vi "test_DAQ_MG090622Camera.vi"() -> ()   [LabVIEW 2010, in "DAQ_MG090622Camera.lvclass"]
uses:
  DAQ_MG090622Camera.lvclass
  GenericDAQ/GenericDAQ/GenericDAQ.lvclass
  main/labview_source/type_definitions/enumerations/run_mode_enum.ctl
  main/labview_source/type_definitions/clusters/controls_refs.ctl
  common/classes/ErrorController/ErrorController/ErrorController.lvclass
panel:
  out "error controller loaded?":bool
  in  "user":string(combo)
  in  "duration":dbl[unit]=1.0
  in  "run mode":T1
  in  "start button":bool
  in  "createButton":bool
  in  "configuration name":string(combo)
  in  "stop":bool
  # "Test Suite for DAQ_MG090622Camera"
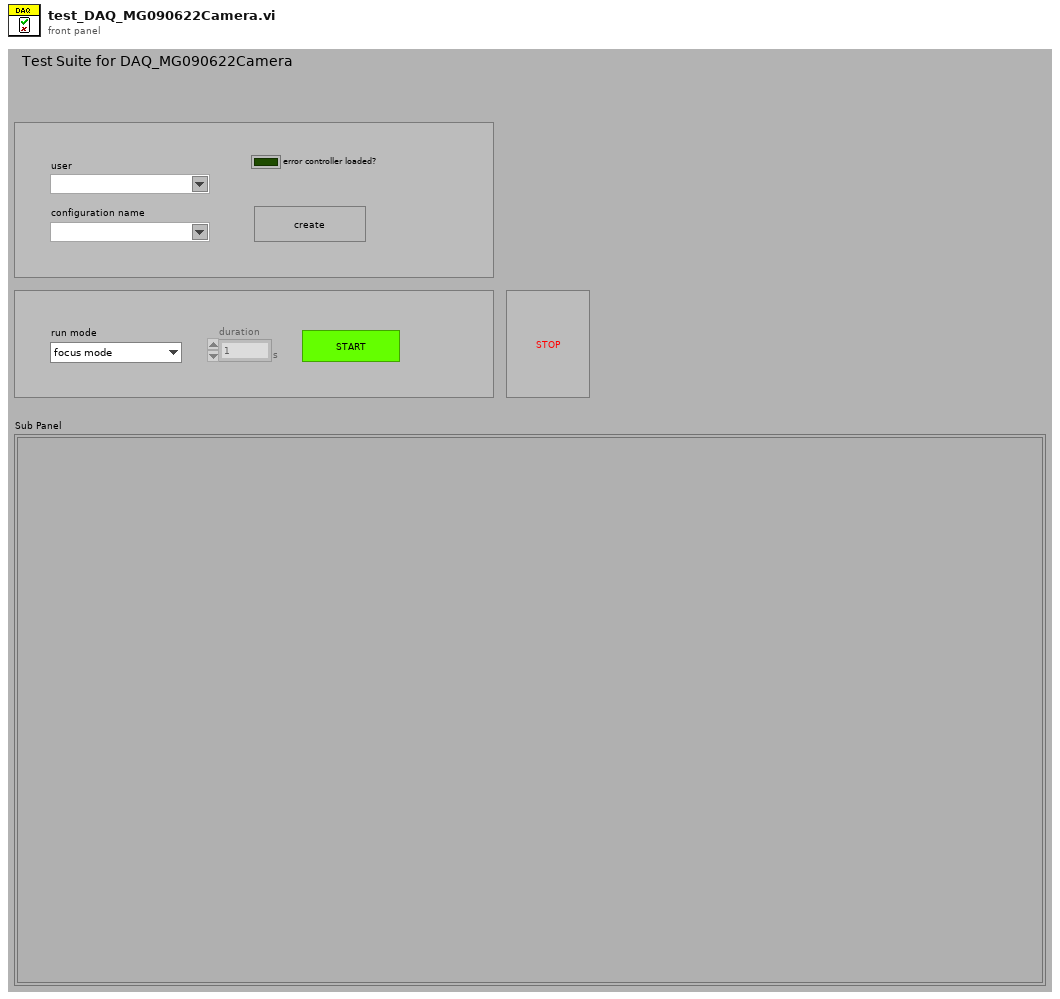
[diagram p1: front panel]
types:
  T1 = typedef "run_mode_enum.ctl" = enum16{"focus mode", "single sweep mode", "experiment mode"}
  T2 = typedef "controls_refs.ctl" = cluster{"scan start button":refnum<vi>, "tabs":cluster{"main":refnum<vi>, "settings":refnum<vi>}, "subpanels":cluster{"imagingMode":refnum<vi>, "scanHead":refnum<vi>, "display":refnum<vi>, "experimentController":refnum<vi>, "instrument":refnum<vi>, "stage":refnum<vi>, "stimulator":refnum<vi>, "dataCollection":refnum<vi>, "analyser":refnum<vi>, "daq":refnum<vi>, "imageAssembler":refnum<vi>}, "drop-downs":cluster{"run mode":refnum<vi>, "imagingMode":refnum<vi>, "experimentalController":refnum<vi>, "objective":refnum<vi>}, "status lights":cluster{"experimentController":refnum<vi>, "imagingMode":refnum<vi>, "scanHead":refnum<vi>, "daq":refnum<vi>, "imageAssembler":refnum<vi>, "dataCollection":refnum<vi>, "display":refnum<vi>, "analyser":refnum<vi>, "stage":refnum<vi>, "stimulator":refnum<vi>, "instrument":refnum<vi>}, "message":refnum<vi>, "stimulator enabled?":refnum<vi>, "saving":cluster{"data folder path":refnum<vi>, "file base name":refnum<vi>, "notebook":refnum<vi>}, "progress bar":refnum<vi>, "update icon":refnum<vi>, "title":refnum<vi>, "main vi":refnum<vi>, "user":refnum<vi>, "exit_button":refnum<vi>, "CPU usage %":refnum<vi>}
  T3 = typedef "plugin_specification.ctl" = cluster{"class path":string, "configuration":string, "label":string, "settings name":string}
  T4 = typedef "GenericToplevelComponent.lvclass/common_trigger_enum.ctl" = enum16{"NULL", "initialise", "terminate", "fetch command", "fetch data", "attach observer", "register as observer", "detach observer", "acknowledge", "start", "stop", "sweep started", "sweep finished", "experiment started", "experiment stopped"}
  T5 = enum8{"Enabled", "Disabled", "Disabled and Grayed Out"}
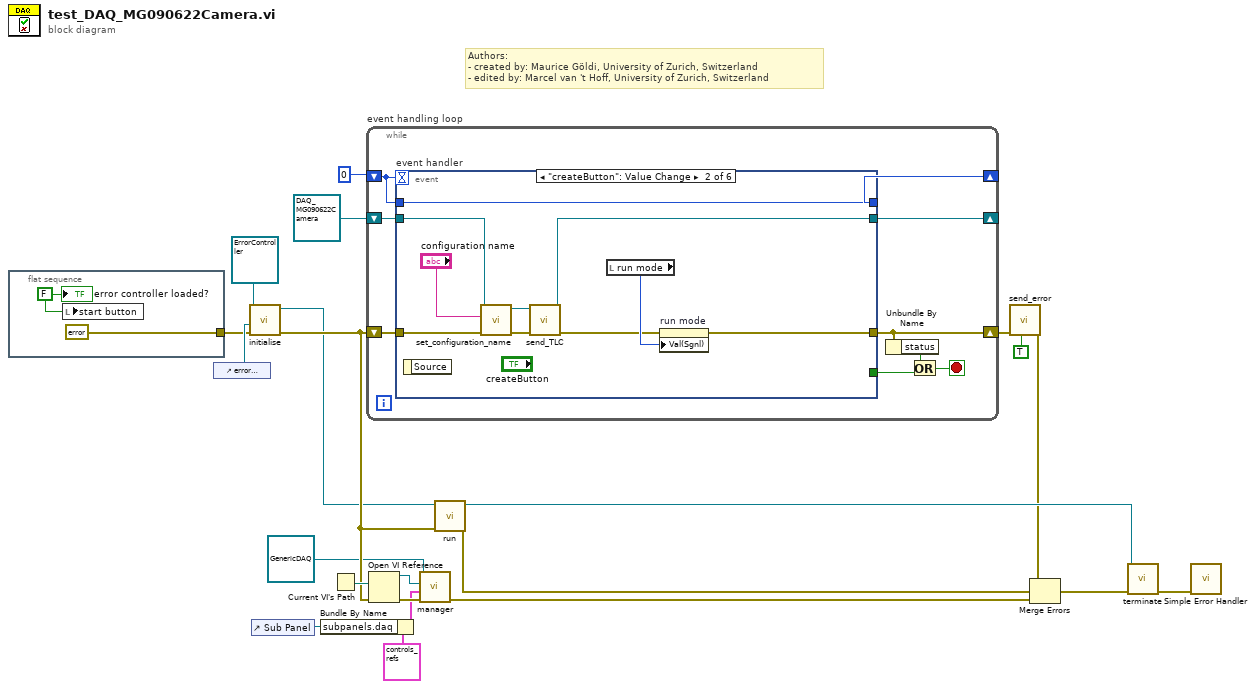
[diagram p0: block diagram]
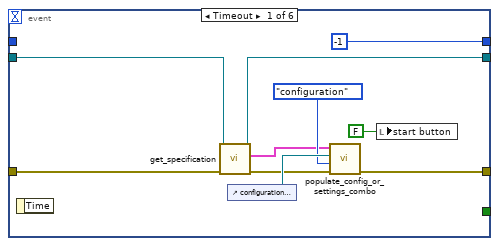
[diagram p2: hidden frame]
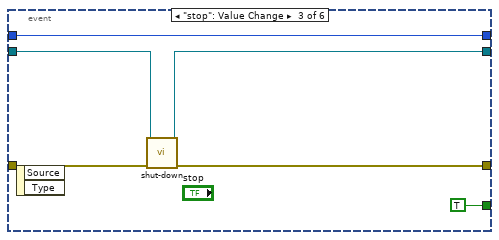
[diagram p3: hidden frame]
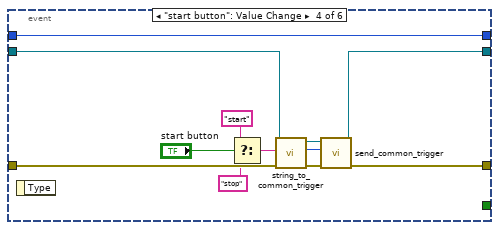
[diagram p4: hidden frame]
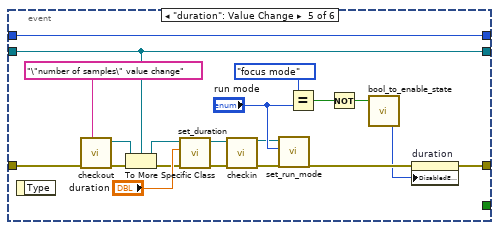
[diagram p5: hidden frame]
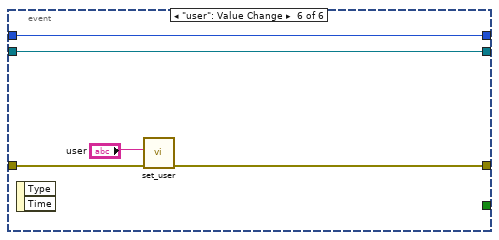
[diagram p6: hidden frame]
diagram:
  # "Authors: \n- created by: Maurice Göldi, University of Zurich, Switzerland\n- edited by: Marcel van 't Hoff, University of Zurich, Switzerland"
  n1 = flat-sequence {
    tunnel: [errorcluster {"status"=FALSE, "code"=0, "source"=""} ("error in (no error)")] -> w2
    frame #0 {
      w23 = FALSE ("error controller loaded?")
      n2 = local write "start button"(w23) -> ()
      "error controller loaded?" <- w23
    }
  }
  n3 = control-ref of="error controller loaded?"() -> (w7:refnum<vi>)
  n4 = call-dynamic "initialise.vi"("error in (no error)"=w2, "error boolean"=w7, "ErrorController in"=refnum<class "ErrorController.lvclass"> refnum) -> ("error out"=w13:errorcluster, "ErrorController out"=w12:refnum<class "ErrorController.lvclass">)  [unwired: 7 in]
  n5 = control-ref of="Sub Panel"() -> (w16:refnum<vi>)
  n6 = Bundle By Name(cluster=T2 {"scan start button"=refnum, "tabs"={"main"=refnum, "settings"=refnum}, "subpanels"={"imagingMode"=refnum, "scanHead"=refnum, "display"=refnum, "experimentController"=refnum, "instrument"=refnum, "stage"=refnum, "stimulator"=refnum, "dataCollection"=refnum, "analyser"=refnum, "daq"=refnum, "imageAssembler"=refnum}, "drop-downs"={"run mode"=refnum, "imagingMode"=refnum, "experimentalController"=refnum, "objective"=refnum}, "status lights"={"experimentController"=refnum, "imagingMode"=refnum, "scanHead"=refnum, "daq"=refnum, "imageAssembler"=refnum, "dataCollection"=refnum, "display"=refnum, "analyser"=refnum, "stage"=refnum, "stimulator"=refnum, "instrument"=refnum}, "message"=refnum, "stimulator enabled?"=refnum, "saving"={"data folder path"=refnum, "file base name"=refnum, "notebook"=refnum}, "progress bar"=refnum, "update icon"=refnum, "title"=refnum, "main vi"=refnum, "user"=refnum, "exit_button"=refnum, "CPU usage %"=refnum} ("control references"), "subpanels.daq"=w16) -> (w15:T2)
  n7 = Current VI's Path() -> (path=w20:path)
  n8 = while "event handling loop" {
    shift-right: [w32] -> _
    shift-left: 0 -> [w33]
    shift-right: [w30] -> _
    shift-left: refnum<class "DAQ_MG090622Camera.lvclass"> refnum ("MG090622IMAQCamera.lvclass") -> [w29]
    shift-right: [w28] -> w4
    shift-left: w13 -> [w31]
    stop <- w25 stop-if-true
    n9 = event "event handler" shown="[1] \"createButton\": Value Change" {
      selector: _ -> [_ _ _ _ _ _]
      dyn-events: _ -> [_ _ _ _ _ _]
      timeout: w33 -> [_ _ _ _ _ _]
      tunnel: w33 -> [_ w53 w59 w71 w91 w96]
      tunnel: [-1 w53 w59 w71 w91 w96] -> w32
      tunnel: [_ _ TRUE _ _ _] -> w26
      tunnel: w31 -> [w38 w52 w57 w65 w90 w93]
      tunnel: [w41 w49 w56 w69 w82 w92] -> w28
      tunnel: [w34 w44 w54 w68 w85 w95] -> w30
      tunnel: w29 -> [w35 w51 w55 w67 w85 w95]
      event Timeout {
        n10 = event-data() -> ()  [unwired: 2 out]
        n11 = call-dynamic "get_specification.vi"("error in (no error)"=w38, "GenericPlugin in"=w35) -> ("error out"=w37:errorcluster, "component specification"=w36:T3, "GenericPlugin out"=w34:refnum<class "DAQ_MG090622Camera.lvclass">)  [unwired: 6 in, 1 out]
        n12 = control-ref of="configuration name"() -> (w42:refnum<vi>)
        n13 = call "populate_config_or_settings_combo.vi"("error in (no error)"=w37, "type"=enum16{"configuration", "settings"}."configuration", "combo-box reference"=w42, "plug-in specification"=w36) -> ("error out"=w41:errorcluster)  [unwired: 7 in]
        n14 = local write "start button"(FALSE ("start button")) -> ()
      }
      event "createButton": Value Change {
        n15 = event-data() -> ()  [unwired: 2 out]
        n16 = call-dynamic "set_configuration_name.vi"("error in (no error)"=w52, "configuration"="configuration name", "GenericPlugin.lvclass in"=w51) -> ("error out"=w46:errorcluster, "GenericPlugin.lvclass out"=w47:refnum<class "DAQ_MG090622Camera.lvclass">)  [unwired: 7 out]
        n17 = call-dynamic "send_TLC.vi"("error in (no error)"=w46, "GenericToplevelComponent in"=w47) -> ("error out"=w45:errorcluster, "GenericToplevelComponent out"=w44:refnum<class "DAQ_MG090622Camera.lvclass">)  [unwired: 8 in]
        n18 = local read "run mode"() -> (w48:T1)
        n19 = property on="run mode" class="Enum (strict)"(error in=w45, "Val(Sgnl)"=w48) -> (error out=w49:errorcluster)  [unwired: 1 in, 1 out]
      }
      event "stop": Value Change {
        n20 = event-data() -> ()  [unwired: 3 out]
        n21 = call-dynamic "shut-down.vi"("error in (no error)"=w57, "GenericToplevelComponent in"=w55) -> ("error out"=w56:errorcluster, "GenericToplevelComponent out"=w54:refnum<class "DAQ_MG090622Camera.lvclass">)  [unwired: 8 out]
      }
      event "start button": Value Change {
        n22 = event-data() -> ()  [unwired: 2 out]
        n23 = Select(t="start", s="start button", f="stop") -> (s? t:f=w60:string)
        n24 = call-dynamic "string_to_common_trigger.vi"("error in (no error)"=w65, "trigger string"=w60, "GenericToplevelComponent in"=w67) -> ("error out"=w64:errorcluster, "trigger"=w63:T4, "GenericToplevelComponent out"=w66:refnum<class "DAQ_MG090622Camera.lvclass">)  [unwired: 6 in]
        n25 = call-dynamic "send_common_trigger.vi"("error in (no error)"=w64, "trigger"=w63, "GenericToplevelComponent in"=w66) -> ("error out"=w69:errorcluster, "GenericToplevelComponent out"=w68:refnum<class "DAQ_MG090622Camera.lvclass">)  [unwired: 6 in, 1 out]
      }
      event "duration": Value Change {
        n26 = event-data() -> ()  [unwired: 2 out]
        n27 = call "checkout.vi"("locked by?"="\"number of samples\" value change", "error in (no error)"=w90) -> ("error out"=w87:errorcluster, "GenericDAQ out"=w84:refnum<class "GenericDAQ.lvclass">)  [unwired: 8 out]
        n28 = To More Specific Class(target class=w85, reference=w84, error in=w87) -> (specific class reference=w83:refnum<class "DAQ_MG090622Camera.lvclass">, error out=w86:errorcluster)
        n29 = call-dynamic "set_duration.vi"("error in (no error)"=w86, "duration"="duration", "DAQ_MG090622Camera in"=w83) -> ("error out"=w79:errorcluster, "DAQ_MG090622Camera out"=w78:refnum<class "DAQ_MG090622Camera.lvclass">)  [unwired: 7 in]
        n30 = call-dynamic "checkin.vi"("error in (no error)"=w79, "GenericDAQ in"=w78) -> ("error out"=w76:errorcluster, "GenericDAQ out"=w77:refnum<class "DAQ_MG090622Camera.lvclass">)  [unwired: 8 in]
        n31 = call-dynamic "set_run_mode.vi"("error in (no error)"=w76, "run mode"="run mode", "GenericPlugin in"=w77) -> ("error out"=w75:errorcluster)  [unwired: 8 out]
        n32 = Equal?(x=run_mode_enum."focus mode" ("run mode"), y="run mode") -> (x = y?=w74:bool)
        n33 = Not(x=w74) -> (.not. x?=w72:bool)
        n34 = call "bool_to_enable_state.vi"("boolean in"=w72) -> ("enabled status out"=w73:T5)  [unwired: 4 in]
        n35 = property on="duration" class="DigNum (strict)"(error in=w75, "DisabledEnum"=w73) -> (error out=w82:errorcluster)  [unwired: 1 in, 1 out]
      }
      event "user": Value Change {
        n36 = event-data() -> ()  [unwired: 3 out]
        n37 = call "set_user.vi"("error in (no error)"=w93, "username in"="user") -> ("error out"=w92:errorcluster)  [unwired: 9 in]
      }
    }
    n38 = Unbundle By Name(w28) -> ("status"=w27:bool)
    n39 = Or(x=w27, y=w26) -> (x .or. y?=w25:bool)
  }
  n40 = Open VI Reference(vi path=w20, error in (no error)=w13) -> (vi reference=w19:refnum<vi>, error out=w18:errorcluster)  [unwired: 4 in]
  n41 = call-dynamic "manager.vi"("error in (no error)"=w18, "control references"=w15, "top-level VI ref in"=w19, "GenericToplevelComponent in"=refnum<class "GenericDAQ.lvclass"> refnum ("GenericDAQ.lvclass")) -> ("error out"=w21:errorcluster)  [unwired: 5 in, 2 out]
  n42 = call "run.vi"("error in (no error)"=w13, "ErrorController in"=w12) -> ("error out"=w11:errorcluster, "ErrorController out"=w9:refnum<class "ErrorController.lvclass">)  [unwired: 8 in]
  n43 = call "send_error.vi"("last error? (F)"=TRUE, "error in (no error)"=w4) -> ("error out"=w5:errorcluster)  [unwired: 9 in]
  n44 = Merge Errors(w5, w11, w21) -> (w6:errorcluster)
  n45 = call-dynamic "terminate.vi"("error in (no error)"=w6, "ErrorController in"=w9) -> ("error out"=w10:errorcluster)  [unwired: 8 in, 1 out]
  n46 = call <vilib>:"Simple Error Handler.vi"("error in (no error)"=w10) -> ()  [unwired: 1 in, 8 out]
